vi "enable.vi"(7 "LVWSR":refnum<class "Web Request.lvclass">, 9 "heater":string, 10 "instr":string, 11 "val":u8) -> ()   [LabVIEW 2017]
uses:
  <vilib>/wsapi/Web Request.lvclass
  Controller/Messages/Enable Heater v MSG/Enable Heater MSG.lvclass
  C:/Program Files (x86)/National Instruments/LabVIEW 2017/vi.lib/ActorFramework/Message/Message.lvclass
  <vilib>/ActorFramework/Message Enqueuer/Message Enqueuer.lvclass/Message Enqueuer.ctl
  <vilib>/ActorFramework/Message Priority Queue/Priority Enqueue.vi
  Controller/gController.lvclass
  <vilib>/ActorFramework/Message Enqueuer/Message Enqueuer.lvclass
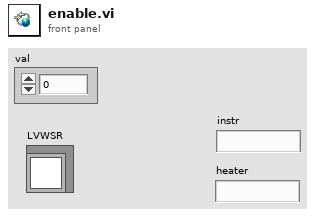
[diagram p1: front panel]
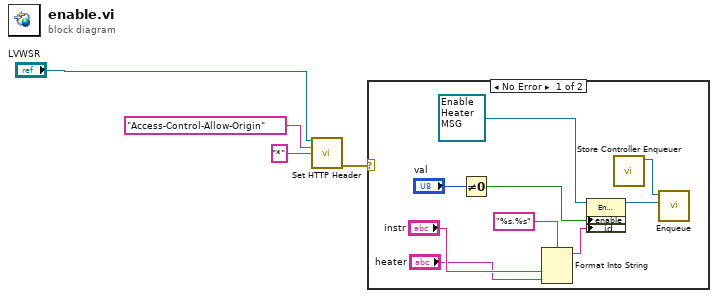
[diagram p0: block diagram]
diagram:
  n1 = call <vilib>:"Set HTTP Header.vi"("LabVIEW Web Service Request"="LVWSR", "header"="Access-Control-Allow-Origin", "header value"="*") -> ("error out"=w2:errorcluster)  [unwired: 11 in, 1 out]
  n2 = case shown="No Error" w2 {
    frame No Error {
      n3 = Not Equal To 0?(x="val") -> (x != 0?=w5:bool)
      n4 = Format Into String(format string="%s.%s", "instr", "heater") -> (resulting string=w11:string)  [unwired: 2 in, 1 out]
      n5 = property class="Enable Heater MSG"(reference=refnum<class "Enable Heater MSG.lvclass"> refnum ("Controller.lvlib:Enable Heater MSG"), "enable"=w5, "id"=w11) -> (reference out=w12:refnum<class "Enable Heater MSG.lvclass">)  [unwired: 1 in, 1 out]
      n6 = call "Store Controller Enqueuer.vi"() -> ("Controller Enqueuer Out"=w13:refnum<class "Message Enqueuer.lvclass">)  [unwired: 11 in]
      n7 = call <vilib>:"Enqueue.vi"("Message"=w12, "Message Enqueuer in"=w13) -> ()  [unwired: 8 in, 2 out]
    }
    frame Error {
    }
  }
